vi "Send CMD.vi"(8 "error in":errorcluster, 10 "CMD In":string, 11 "Vaisala in":refnum<class "FPGA Vaisala.lvclass">) -> (0 "error out":errorcluster, 3 "Vaisala out":refnum<class "FPGA Vaisala.lvclass">)   [LabVIEW 2014, in "FPGA Vaisala.lvclass"]
uses:
  FPGA Vaisala.lvclass
  <vilib>/rvi/interface/nirviReadWriteControl/nirviReadWriteControl.xnode
  Instruments/Nicholas/FPGA/RS485 In.ctl
  <vilib>/rvi/interface/nirviMethod/nirviMethod.xnode
  <vilib>/rvi/errors/niLvFpgaMergeErrorWithErrorCode.vi
  <vilib>/rvi/errors/niLvFpgaAdjustHostInterfaceError.vi
  <vilib>/FPGAPlugInAG/cRIO-9081/niLvFpga_AcknowledgeIrq_cRIO-9081.vi
  <vilib>/rvi/interface/nirviMethod/StockFPGA_InlinedMethodWaitForSingleIRQ.vi
  <vilib>/FPGAPlugInAG/cRIO-9081/niLvFpga_WaitOnIrq_cRIO-9081.vi
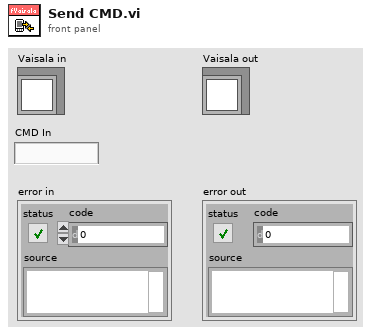
[diagram p1: front panel]
types:
  T1 = enum16{"Port 1", "Port 2", "Port 3", "Port 4", "None"}
  T2 = typedef "RS485 In.ctl" = cluster{"Data":u8[], "NumBytes":i32, "RS485_Cmd":enum16{"Read", "Write", "Idle"}, "New":bool, "Port":enum16{"Port 1", "Port 2", "Port 3", "Port 4", "None"}, "Timeout (ms)":i32}
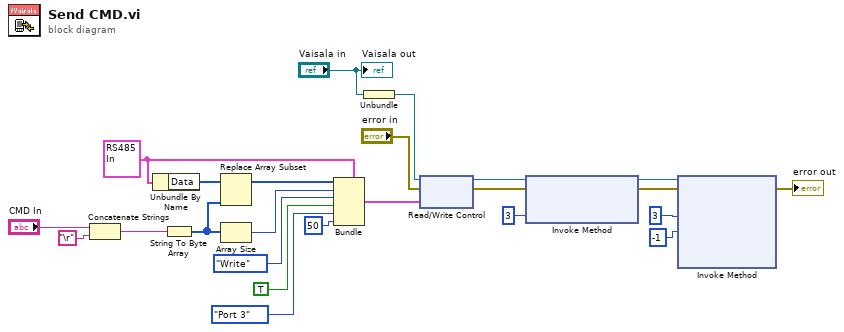
[diagram p0: block diagram]
diagram:
  w22 = T2 {"Data"=[0, 0, 0, 0, 0, 0, 0, 0, 0, 0, 0, 0, 0, 0, 0, 0, 0, 0, 0, 0, 0, 0, 0, 0, 0, 0, 0, 0, 0, 0, 0, 0, 0, 0, 0, 0, 0, 0, 0, 0, 0, 0, 0, 0, 0, 0, 0, 0, 0, 0, 0, 0, 0, 0, 0, 0, 0, 0, 0, 0, 0, 0, 0, 0, 0, 0, 0, 0, 0, 0, 0, 0, 0, 0, 0, 0, 0, 0, 0, 0, 0, 0, 0, 0, 0, 0, 0, 0, 0, 0, 0, 0, 0, 0, 0, 0, 0, 0, 0, 0], "NumBytes"=0, "RS485_Cmd"=enum."Write", "New"=FALSE, "Port"=enum."Port 1", "Timeout (ms)"=0} ("Input")
  n1 = Concatenate Strings("CMD In", "\r") -> (w23:string)
  n2 = Unbundle By Name(w22) -> ("Data"=w20:u8[])
  n3 = String To Byte Array(string=w23) -> (unsigned byte array=w19:u8[])
  n4 = Replace Array Subset(array=w20, new element=w19) -> (w18:u8[])  [unwired: 1 in]
  n5 = Array Size(array=w19) -> (size(s)=w24:i32)
  n6 = Bundle(cluster=w22, "Data"=w18, "NumBytes"=w24, "RS485_Cmd"=enum16{"Read", "Write", "Idle"}."Write", "New"=TRUE ("New Message"), "Port"=T1."Port 3", "Timeout (ms)"=50) -> (w17:T2)
  n7 = Unbundle("Vaisala in") -> (w14:refnum<k20>)
  n8 = xnode "Read/Write Control"("FPGA VI Reference In"=w14, "error in"="error in", "Input"=w17) -> ("FPGA VI Reference Out"=w4:refnum<k20>, "error out"=w2:errorcluster)
  n9 = xnode "Invoke Method"("FPGA VI Reference In"=w4, "error in"=w2, "IRQ Number(s)"=3) -> ("FPGA VI Reference Out"=w8:refnum<k20>, "error out"=w7:errorcluster)
  n10 = xnode "Invoke Method"("FPGA VI Reference In"=w8, "error in"=w7, "IRQ Number(s)"=3, "Timeout (ms)"=-1) -> ("error out"=→"error out":errorcluster)  [unwired: 3 out]
  "Vaisala out" <- "Vaisala in"
